vi "FS Sketch.vi"   [LabVIEW 2019]
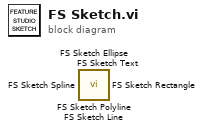
[diagram p0: block diagram]
diagram:
  n1 = call <userlib>:"FS Sketch Polyline.vi"() -> ()  [unwired: 11 in, 1 out]
  n2 = call "FS Sketch Text.vi"() -> ()  [unwired: 11 in, 1 out]
  n3 = call <userlib>:"FS Sketch Spline.vi"() -> ()  [unwired: 11 in, 1 out]
  n4 = call <userlib>:"FS Sketch Rectangle.vi"() -> ()  [unwired: 11 in, 1 out]
  n5 = call <userlib>:"FS Sketch Line.vi"() -> ()  [unwired: 11 in, 1 out]
  n6 = call <userlib>:"FS Sketch Ellipse.vi"() -> ()  [unwired: 11 in, 1 out]
